vi "添加图形至集合.vi"(8 "error in (no error)":errorcluster caption="错误输入（无错误）", 10 "图形.lvclass":refnum<class "图形.lvclass">, 11 "集合 输入":refnum<class "集合.lvclass"> caption="DNL_LabVIEW Object in") -> (0 "error out":errorcluster caption="错误输出", 3 "集合 输出":refnum<class "集合.lvclass"> caption="DNL_LabVIEW Object out")   [LabVIEW 2011, in "集合.lvclass"]
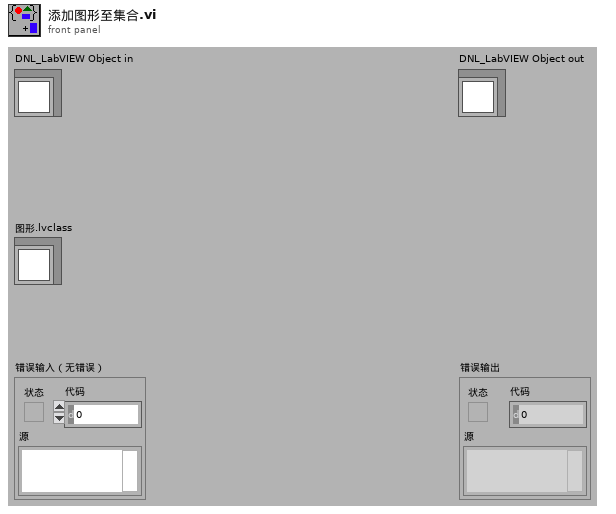
[diagram p1: front panel]
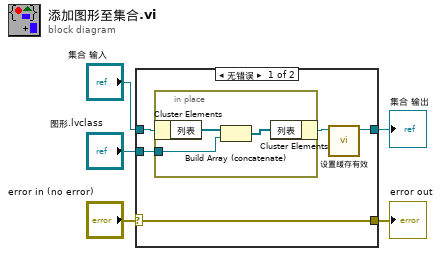
[diagram p0: block diagram]
diagram:
  n1 = case shown="无错误" "error in (no error)" {
    selector: "error in (no error)" -> [w10 w15]
    tunnel: [w10 w15] -> w4
    tunnel: [w6 w14] -> w2
    tunnel: "集合 输入" -> [w9 w14]
    tunnel: "图形.lvclass" -> [w8 _]
    frame No Error {
      n2 = in-place {
        in-place-border: w8 -> [w12]
        n3 = in-place-cluster #1(w9) -> ("列表"=w13:refnum<class "图形.lvclass">[])
        n4 = Build Array (concatenate)(w13, w12) -> (w11:refnum<class "图形.lvclass">[])
        n5 = in-place-cluster #1("列表"=w11) -> (w7:refnum<class "集合.lvclass">)
      }
      n6 = call "设置缓存有效.vi"("图形 输入"=w7) -> ("图形 输出"=w6:refnum<class "集合.lvclass">)  [unwired: 9 in, 1 out]
    }
    frame Error {
    }
  }
  "error out" <- w4
  "集合 输出" <- w2
